vi "Sub_MotorL.vi"(1 "L":i32) -> (0 "문자열":string)   [LabVIEW 2013]
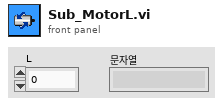
[diagram p1: front panel]
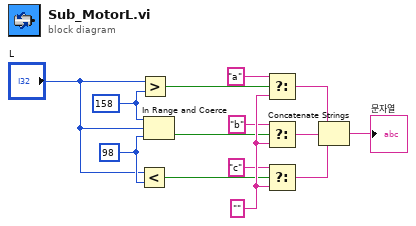
[diagram p0: block diagram]
diagram:
  w14 = ""
  w5 = 98
  w6 = 158
  n1 = Less?(x="L", y=w5) -> (x < y?=w4:bool)
  n2 = Greater?(x="L", y=w6) -> (0:w2:bool)
  n3 = In Range and Coerce(upper limit=w6, x="L", lower limit=w5) -> (In Range?=w3:bool)  [unwired: 1 out]
  n4 = Select(t="a", s=w2, f=w14) -> (s? t:f=w10:string)
  n5 = Select(t="b", s=w3, f=w14) -> (s? t:f=w11:string)
  n6 = Select(t="c", s=w4, f=w14) -> (s? t:f=w12:string)
  n7 = Concatenate Strings(w10, w11, w12) -> (→"문자열":string)
